vi "Desktop Main.vi"() -> ()   [LabVIEW 2018]
uses:
  Controls/Channel Settings.ctl
  Controls/Analog Input Selector.ctl
  Controls/Knob.ctl
  Controls/Vertical Position.ctl
  Controls/Time Selector.ctl
  Controls/Time Knob.ctl
  Controls/Instrument Control.ctl
  Controls/Acquisition Mode.ctl
  Controls/Measurements.ctl
  Controls/Channel Measurement String Control.ctl
  Controls/Options.ctl
  Controls/Channel.ctl
  Controls/Function Generator Control.ctl
  Program Files (x86)/National Instruments/LabVIEW 2018/ProjectTemplates/Source/myRIO/Oscilloscope/myRIO v1.1/Real-Time/Controls/Waveform Enum.ctl
  Program Files (x86)/National Instruments/LabVIEW 2018/ProjectTemplates/Source/myRIO/Oscilloscope/myRIO v1.1/Real-Time/Controls/Channel Selector.ctl
  Controls/Program Data.ctl
  Controls/Cursor Info.ctl
  Controls/Communication Cluster.ctl
  <vilib>/NI/STM/TCP/TCP Connection Info.ctl
  <vilib>/NI/STM/SubVIs/MetaDataElement.ctl
  Communication/Scope Data.ctl
  Program Files (x86)/National Instruments/LabVIEW 2018/ProjectTemplates/Source/myRIO/Oscilloscope/myRIO v1.1/Real-Time/Controls/Wave Parameters.ctl
  Controls/Channel Parameters.ctl
  Controls/FGen Desktop Configuration.ctl
  Controls/Measurement Selector.ctl
  Queue Library/User Event Action Enum.ctl
  Controls/Scope & FGen Parameters.ctl
  Controls/FGen FGV Enum.ctl
  Queue Library/Queue Library.lvlib
  <vilib>/NI/STM/NI STM.lvlib
panel:
  out "Acquiring?":bool
  out "Gen?":bool
  out "Sweep?":bool
  out "Scope Screen":waveform(dbl)[](graph)
  in  "Function Generator":T1 {"Vpeak (V)" min=0.0; "Frequency (Hz)" min=0.0}
  out "error out":errorcluster
  in  "Options":T4={"Enable\nCursors"=FALSE, "C1"=enum."CH 0", "C2"=enum."CH 0", "CH 0"=FALSE, "CH 1"=FALSE, "IP"="172.22.11.2"}
  out "Measurements":T6={"Channel 0"="Channel 0", "RMS 0"="RMS:", "Vp-p 0"="Vp-p:", "Freq 0"="Freq:", "Channel 1"="Channel 1", "RMS 1"="RMS:", "Vp-p 1"="Vp-p:", "Freq 1"="Freq:", "Cursors"="Cursors", "C1"="C1:", "C2"="C2:", "dT"="dT:"}
  in  "Acquisition Control":T8
  in  "Time":T10={"Time/Div"=6.0} {"Time/Div" min=0.0 max=16.0 step=1.0 scale=0.0..12.0}
  in  "Channel 1 Settings":T12={"Channel"=enum."AI 1", "Enable"=FALSE, "Volts/Div"=5, "Vertical Position (Div)"=0.0} {"Vertical Position (Div)" min=-5.0 max=5.0 step=0.1 scale=-5.0..5.0; "Volts/Div" min=0 max=8 step=1 scale=0.0..8.0}
  in  "Channel 0 Settings":T12={"Channel"=enum."AI 0", "Enable"=TRUE, "Volts/Div"=5, "Vertical Position (Div)"=0.0} {"Vertical Position (Div)" min=-5.0 max=5.0 step=0.1 scale=-5.0..5.0; "Volts/Div" min=0 max=8 step=1 scale=0.0..8.0}
  # "Scope & FGen for NI myRIO"
  # "Measurements"
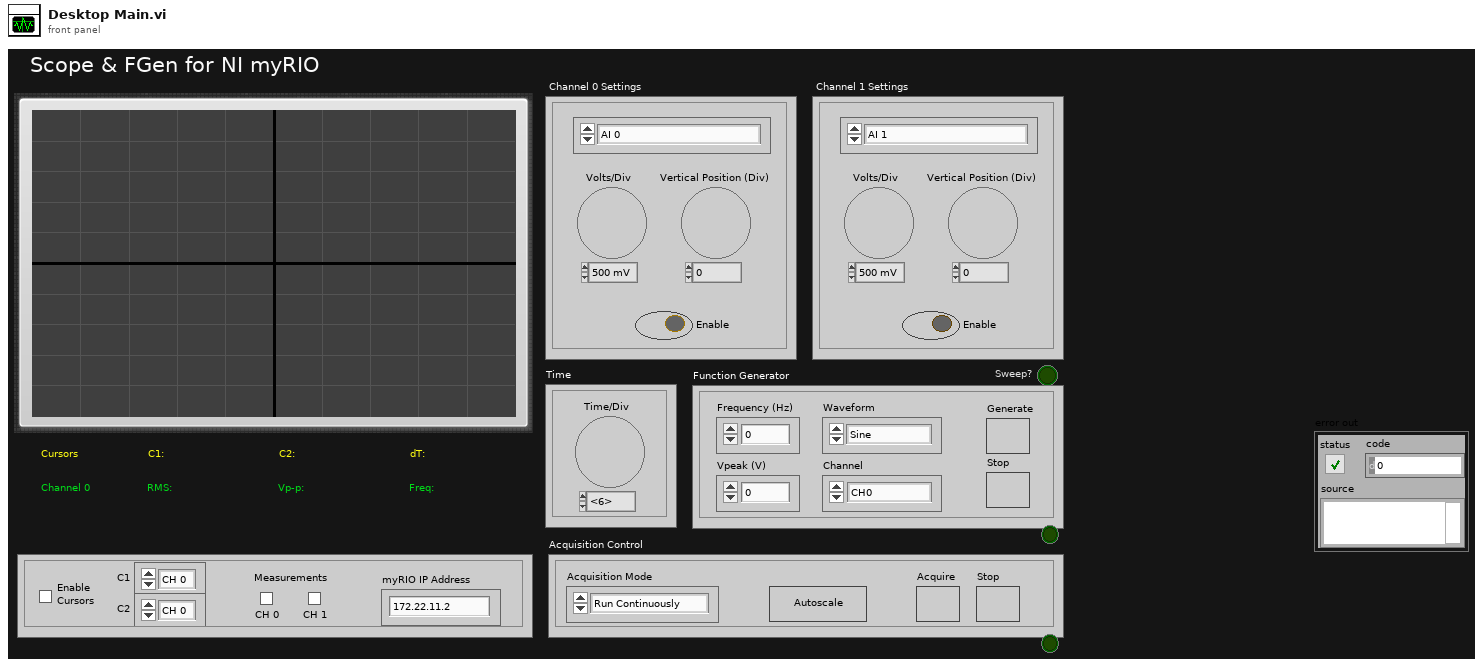
[diagram p1: front panel]
types:
  T1 = typedef "Function Generator Control.ctl" = cluster{"Frequency (Hz)":dbl, "Vpeak (V)":dbl, "Waveform":T2, "Channel":T3, "Generate":bool, "Stop":bool}
  T2 = typedef "Waveform Enum.ctl" = enum16{"Sine", "Square"}
  T3 = typedef "Channel Selector.ctl" = enum16{"CH0", "CH1"}
  T4 = typedef "Options.ctl" = cluster{"Enable\nCursors":bool, "C1":T5, "C2":T5, "CH 0":bool, "CH 1":bool, "IP":string}
  T5 = typedef "Channel.ctl" = enum16{"CH 0", "CH 1"}
  T6 = typedef "Measurements.ctl" = cluster{"Channel 0":T7, "RMS 0":T7, "Vp-p 0":T7, "Freq 0":T7, "Channel 1":T7, "RMS 1":T7, "Vp-p 1":T7, "Freq 1":T7, "Cursors":T7, "C1":T7, "C2":T7, "dT":T7}
  T7 = typedef "Channel Measurement String Control.ctl" = string
  T8 = typedef "Instrument Control.ctl" = cluster{"Acquisition Mode":T9, "Acquire":bool, "Stop":bool, "Autoscale":bool}
  T9 = typedef "Acquisition Mode.ctl" = enum16{"Run Continuously", "Run Once"}
  T10 = typedef "Time Selector.ctl" = cluster{"Time/Div":T11}
  T11 = typedef "Time Knob.ctl" = dbl
  T12 = typedef "Channel Settings.ctl" = cluster{"Channel":T13, "Enable":bool, "Volts/Div":T14, "Vertical Position (Div)":T15}
  T13 = typedef "Analog Input Selector.ctl" = enum16{"AI 0", "AI 1"}
  T14 = typedef "Knob.ctl" = i32
  T15 = typedef "Vertical Position.ctl" = dbl
  T16 = typedef "Queue Library.lvlib/User Event Action Enum.ctl" = enum16{"Initialize", "Generate", "Destroy"}
  T17 = typedef "Measurement Selector.ctl" = enum16{"CH0", "CH1", "Cursors"}
  T18 = typedef "Program Data.ctl" = cluster{"Measurements":T6, "C1":T19, "C2":T19, "Com":T20, "Continuous?":bool, "Scope Data":T23, "Wave Parameters":T24, "Acquire?":bool, "Measure Ref":refnum<vi>, "CH0":T12, "CH1":T12, "CH0 Params":T25, "CH1 Params":T25, "Time":T10, "dT":dbl, "FGen":T26}
  T19 = typedef "Cursor Info.ctl" = cluster{"Name":string, "X":dbl, "Y":dbl}
  T20 = typedef "Communication Cluster.ctl" = cluster{"Connection Info":T21, "Connected?":bool, "IP":string}
  T21 = typedef "NI STM.lvlib/TCP Connection Info.ctl" = cluster{"connection ID":refnum<k5>, "meta data":T22[]}
  T22 = typedef "NI STM.lvlib/MetaDataElement.ctl" = string
  T23 = typedef "Scope Data.ctl" = cluster{"AI0":dbl[], "AI1":dbl[]}
  T24 = typedef "Wave Parameters.ctl" = cluster{"Frequency (Hz)":dbl, "Phase offset (deg)":dbl, "Vpeak (V)":dbl, "Offset (V)":dbl, "Waveform":T2, "Channel":T3}
  T25 = typedef "Channel Parameters.ctl" = cluster{"V/Div":dbl, "Units":string}
  T26 = typedef "FGen Desktop Configuration.ctl" = cluster{"Offset (V)":dbl, "Enable Sweep":bool, "Start Frequency (Hz)":dbl, "Stop Frequency (Hz)":dbl, "Step (Hz)":dbl, "Step Interval (ms)":dbl, "Current Freq (Hz)":dbl, "Run":bool}
  T27 = typedef "FGen FGV Enum.ctl" = enum16{"Set", "Get"}
  T28 = typedef "Scope & FGen Parameters.ctl" = cluster{"Acquire?":bool, "Wave Parameters":T24, "Time":T10}
  T29 = typedef "State.ctl" = enum16{"Initialize", "Idle", "Start Scope", "Acquire", "Stop Scope", "Config FGen", "Start FGen", "Sweep FGen", "Stop FGen", "Plot", "Option Selection", "Channel 0 Selection", "Channel 1 Selection", "Update Cursors", "Update Measurements", "Time/Div", "Autoscale", "Stop", "Error"}
  T30 = cluster{"Cursor.Cursor Name":string, "Cursor.Cursor X":dbl, "Cursor.Cursor Y":dbl}
  T31 = cluster{"Cursor Name":string, "Cursor X":dbl, "Cursor Y":dbl}
  T32 = cluster{"Enable\nCursors":bool, "C1":bool, "C2":bool, "CH 0":bool, "CH 1":bool, "IP":bool}
  T33 = cluster{"Channel":bool, "Enable":bool, "Volts/Div":bool, "Vertical Position (Div)":bool}
  T34 = cluster{"Acquisition Mode":bool, "Acquire":bool, "Stop":bool, "Autoscale":bool}
  T35 = cluster{"Frequency (Hz)":bool, "Vpeak (V)":bool, "Waveform":bool, "Channel":bool, "Generate":bool, "Stop":bool}
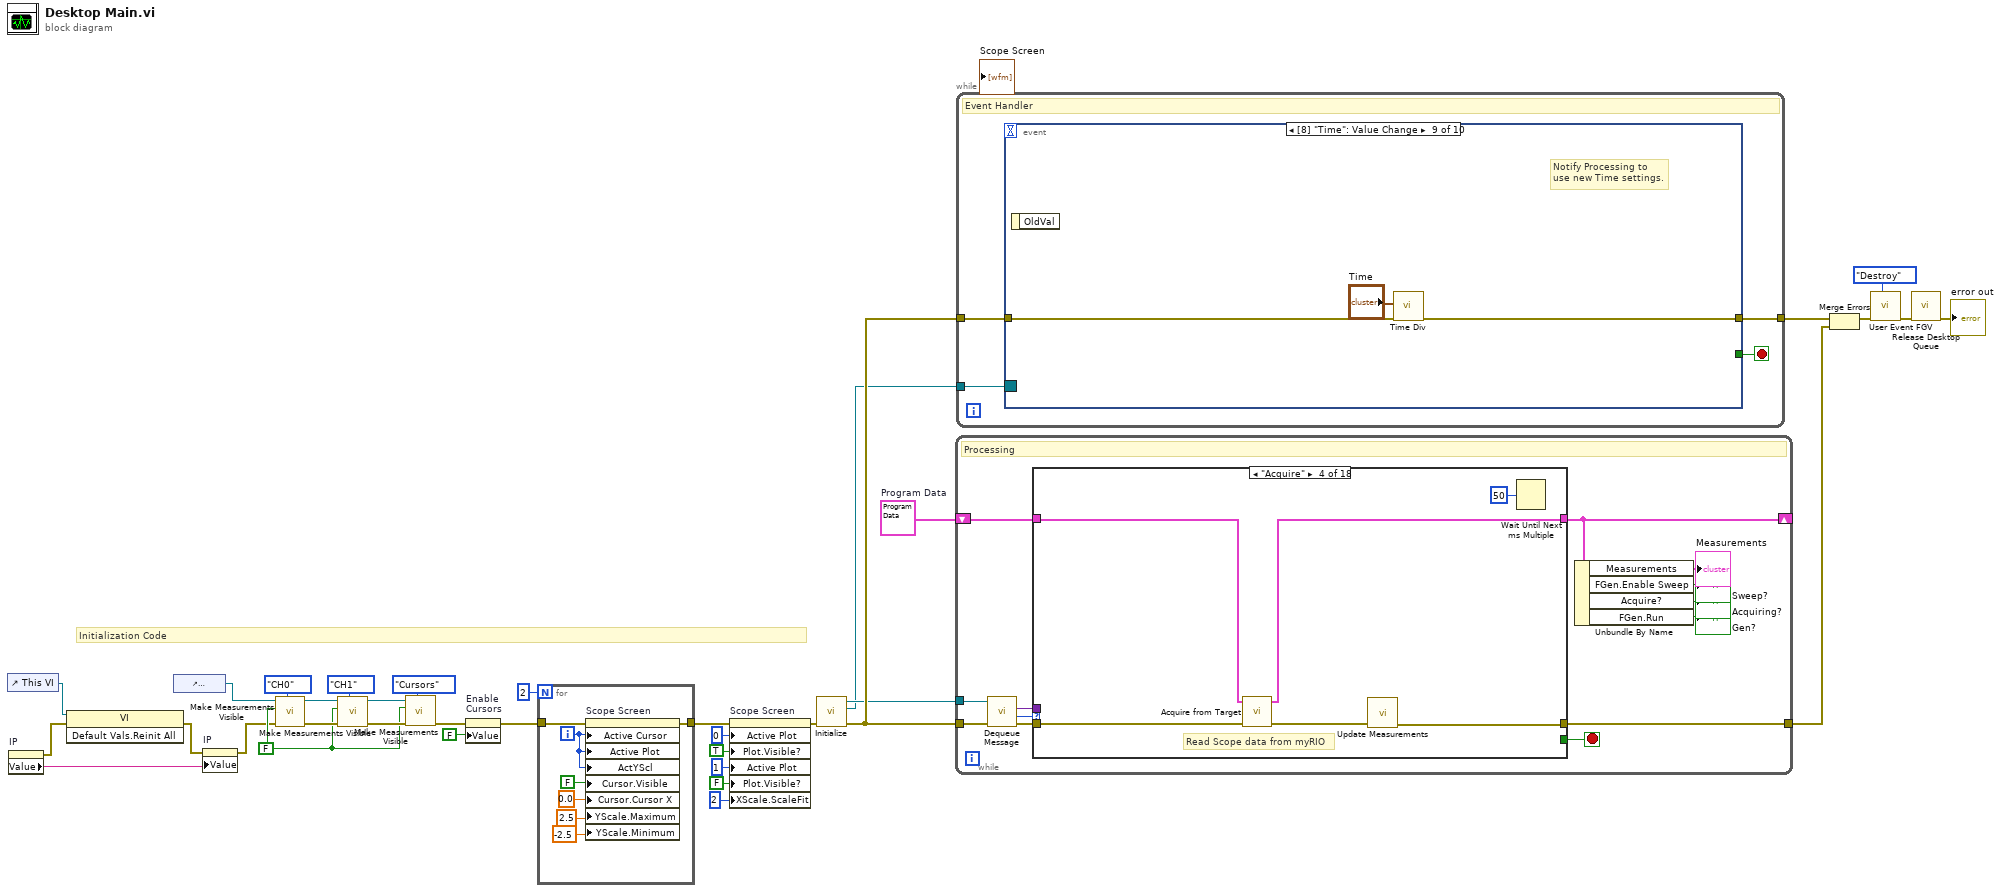
[diagram p0: block diagram]
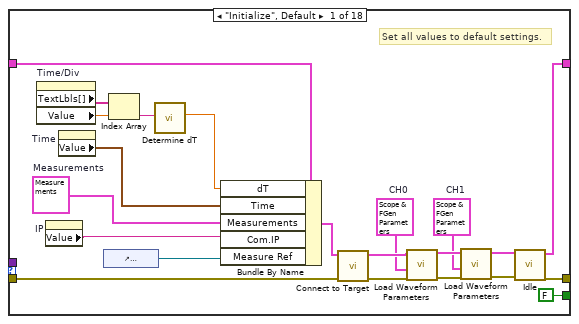
[diagram p2: hidden frame]
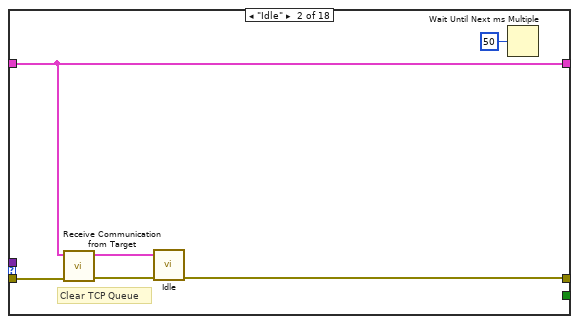
[diagram p3: hidden frame]
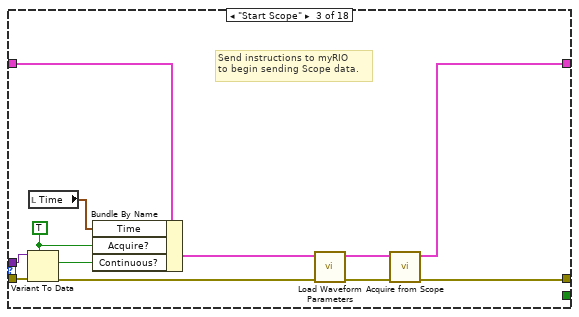
[diagram p4: hidden frame]
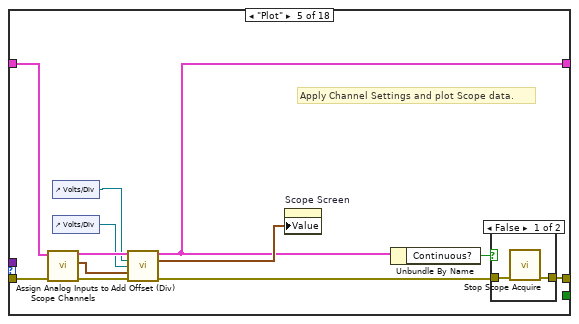
[diagram p5: hidden frame]
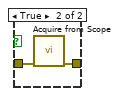
[diagram p6: hidden frame]
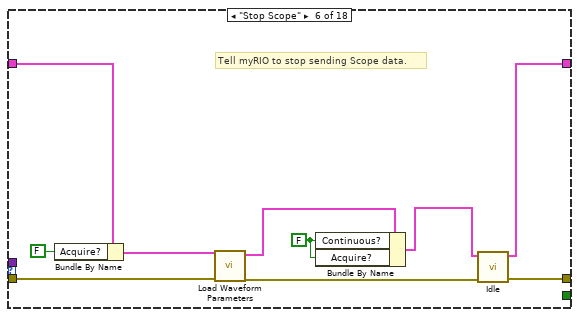
[diagram p7: hidden frame]
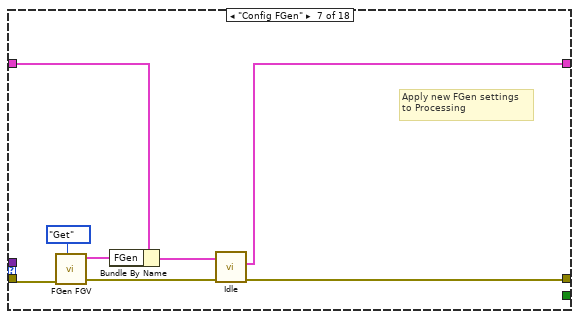
[diagram p8: hidden frame]
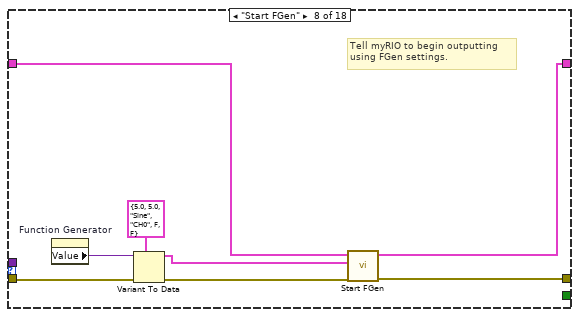
[diagram p9: hidden frame]
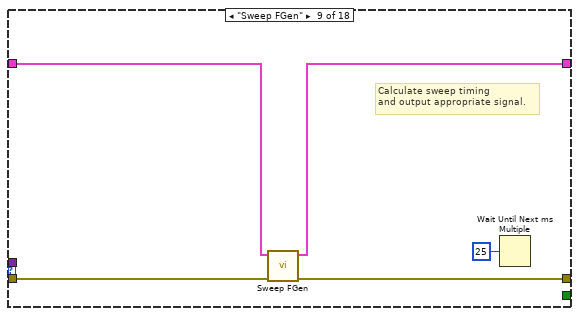
[diagram p10: hidden frame]
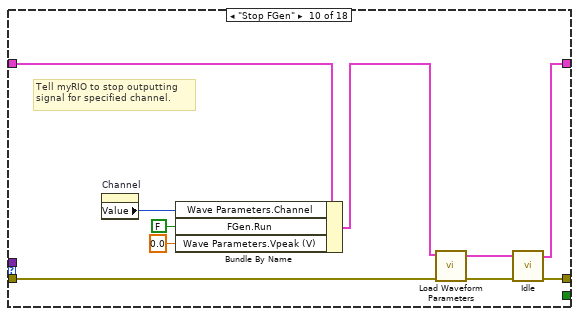
[diagram p11: hidden frame]
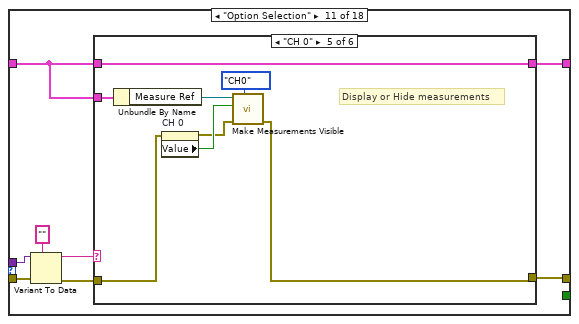
[diagram p12: hidden frame]
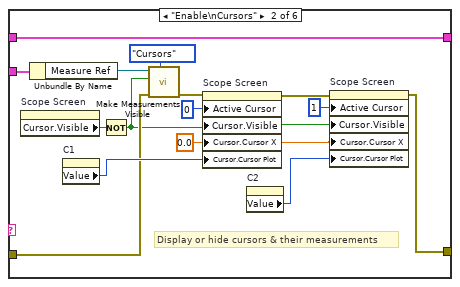
[diagram p14: hidden frame]
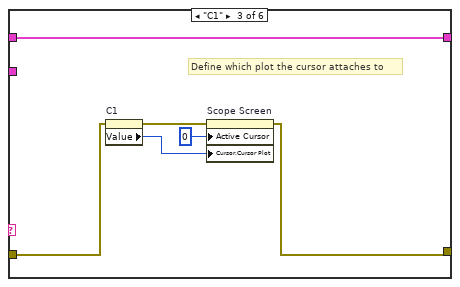
[diagram p15: hidden frame]
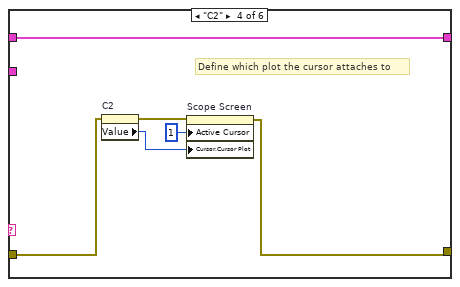
[diagram p16: hidden frame]
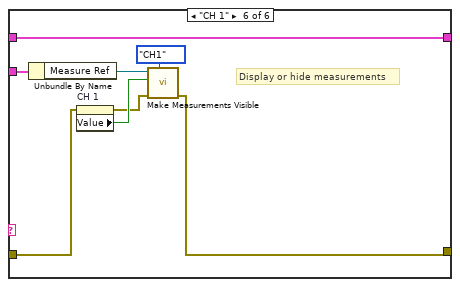
[diagram p17: hidden frame]
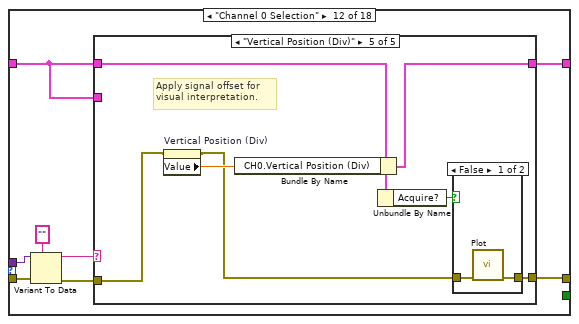
[diagram p18: hidden frame]
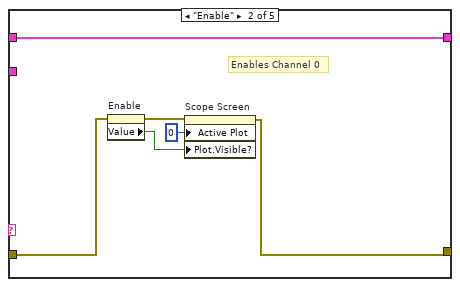
[diagram p20: hidden frame]
diagram:
  w17 = FALSE ("Visible?")
  w31 = T18 {"Measurements"={"Channel 0"="", "RMS 0"="", "Vp-p 0"="", "Freq 0"="", "Channel 1"="", "RMS 1"="", "Vp-p 1"="", "Freq 1"="", "Cursors"="", "C1"="", "C2"="", "dT"=""}, "C1"={"Name"="", "X"=0.0, "Y"=0.0}, "C2"={"Name"="", "X"=0.0, "Y"=0.0}, "Com"={"Connection Info"={"connection ID"=refnum, "meta data"=[]}, "Connected?"=FALSE, "IP"=""}, "Continuous?"=FALSE, "Scope Data"={"AI0"=[], "AI1"=[]}, "Wave Parameters"={"Frequency (Hz)"=0.0, "Phase offset (deg)"=0.0, "Vpeak (V)"=0.0, "Offset (V)"=0.0, "Waveform"=enum."Sine", "Channel"=enum."CH0"}, "Acquire?"=FALSE, "Measure Ref"=refnum, "CH0"={"Channel"=enum."AI 0", "Enable"=TRUE, "Volts/Div"=5, "Vertical Position (Div)"=0.0}, "CH1"={"Channel"=enum."AI 1", "Enable"=FALSE, "Volts/Div"=5, "Vertical Position (Div)"=0.0}, "CH0 Params"={"V/Div"=0.5, "Units"="V"}, "CH1 Params"={"V/Div"=0.5, "Units"="V"}, "Time"={"Time/Div"=0.0}, "dT"=0.0, "FGen"={"Offset (V)"=0.0, "Enable Sweep"=FALSE, "Start Frequency (Hz)"=0.0, "Stop Frequency (Hz)"=0.0, "Step (Hz)"=0.0, "Step Interval (ms)"=0.0, "Current Freq (Hz)"=0.0, "Run"=FALSE}}  # Program Data
  # "Initialization Code"
  n1 = control-ref of="This VI"() -> (w24:refnum<vi>)
  n2 = property on="IP" class="Str"() -> (error out=w2:errorcluster, "Value"=w1:string)  [unwired: 2 in, 1 out]
  n3 = invoke class="VI" method="Default Vals.Reinit All"(reference=w24, error in=w2) -> (error out=w4:errorcluster)  [unwired: 1 in, 2 out]
  n4 = control-ref of="Measurements"() -> (w16:refnum<vi>)
  n5 = property on="IP" class="Str"(error in=w4, "Value"=w1) -> (error out=w3:errorcluster)  [unwired: 1 in, 1 out]
  n6 = call "Make Measurements Visible.vi"("Item"=Measurement_Selector."CH0", "error in (no error)"=w3, "Visible?"=w17, "Measurements Ref"=w16) -> ("error out"=w23:errorcluster)  [unwired: 7 in]
  n7 = call "Make Measurements Visible.vi"("Item"=Measurement_Selector."CH1", "error in (no error)"=w23, "Visible?"=w17, "Measurements Ref"=w16) -> ("error out"=w20:errorcluster)  [unwired: 7 in]
  n8 = call "Make Measurements Visible.vi"("Item"=Measurement_Selector."Cursors", "error in (no error)"=w20, "Visible?"=w17, "Measurements Ref"=w16) -> ("error out"=w19:errorcluster)  [unwired: 7 in]
  n9 = property on="Enable\nCursors" class="Bool (strict)"(error in=w19, "Value"=FALSE) -> (error out=w25:errorcluster)  [unwired: 1 in, 1 out]
  n10 = for {
    N: 2 -> [_]
    tunnel: w25 -> [w38]
    tunnel: [w37] -> w11
    i -> [w36]
    n11 = property on="Scope Screen" class="WFGraph (strict)"(error in=w38, "Active Cursor"=w36, "Active Plot"=w36, "ActYScl"=w36, "Cursor.Visible"=FALSE, "Cursor.Cursor X"=0.0 ("Cursor.Cursor Position:Cursor X"), "YScale.Maximum"=2.5 ("Y Scale.Range:Maximum"), "YScale.Minimum"=-2.5 ("Y Scale.Range:Minimum")) -> (error out=w37:errorcluster)  [unwired: 1 in, 1 out]
  }
  n12 = property on="Scope Screen" class="WFGraph (strict)"(error in=w11, "Active Plot"=u32 0, "Plot.Visible?"=TRUE ("Plot.Visible"), "Active Plot"=u32 1, "Plot.Visible?"=FALSE ("Plot.Visible"), "XScale.ScaleFit"=u8 2 ("X Scale.Scale Fit")) -> (error out=w6:errorcluster)  [unwired: 1 in, 1 out]
  n13 = call "Initialize.vi"("error in (no error)"=w6) -> ("error out"=w30:errorcluster, "User Event Out"=w10:refnum<event-registration>, "queue out"=w29:refnum<queue>)  [unwired: 8 in]
  n14 = while {
    tunnel: w29 -> [w43]
    tunnel: w30 -> [w53]
    tunnel: [w48] -> w32
    shift-right: [w46] -> _
    shift-left: w31 -> [w47]
    stop <- w50 stop-if-true
    # "Processing"
    n15 = call "Dequeue Message.vi"("error in (no error)"=w53, "queue in"=w43) -> ("error out"=w49:errorcluster, "State"=w52:T29, "Data"=w51:variant)  [unwired: 6 in, 1 out]
    n16 = case shown="\"Acquire\"" w52 {
      tunnel: w51 -> [_ _ w91 _ _ _ _ _ _ _ w162 w215 w260 _ w333 w346 _ _]
      tunnel: [FALSE _ _ _ _ _ _ _ _ _ _ _ _ FALSE FALSE _ _ TRUE] -> w50
      tunnel: w49 -> [w72 w81 w92 w97 w107 w123 w131 w140 w145 w153 w163 w216 w261 w306 w334 w347 w380 w391]
      tunnel: [w67 w78 w86 w93 w110 w118 w125 w139 w143 w155 w158 w211 w256 w311 w327 w341 w377 w388] -> w48
      tunnel: w47 -> [w74 w80 w84 w96 w108 w121 w132 w133 w144 w152 w157 w210 w255 w308 w330 w338 w379 w387]
      tunnel: [w66 w80 w90 w95 w101 w115 w126 w138 w142 w148 w156 w209 w254 w300 w329 w339 w375 w386] -> w46
      frame "Initialize", Default {
        w54 = T28 {"Acquire?"=FALSE, "Wave Parameters"={"Frequency (Hz)"=0.0, "Phase offset (deg)"=0.0, "Vpeak (V)"=0.0, "Offset (V)"=0.0, "Waveform"=enum."Sine", "Channel"=enum."CH1"}, "Time"={"Time/Div"=9.0}}  # CH1
        w68 = T28 {"Acquire?"=FALSE, "Wave Parameters"={"Frequency (Hz)"=0.0, "Phase offset (deg)"=0.0, "Vpeak (V)"=0.0, "Offset (V)"=0.0, "Waveform"=enum."Sine", "Channel"=enum."CH0"}, "Time"={"Time/Div"=9.0}}  # CH0
        w73 = T6 {"Channel 0"="Channel 0", "RMS 0"="RMS:", "Vp-p 0"="Vp-p:", "Freq 0"="Freq:", "Channel 1"="Channel 1", "RMS 1"="RMS:", "Vp-p 1"="Vp-p:", "Freq 1"="Freq:", "Cursors"="Cursors", "C1"="C1:", "C2"="C2:", "dT"="dT:"}  # Measurements
        # "Set all values to default settings."
        n17 = property on="Time/Div" class="Knob (strict)"() -> ("TextLbls[]"=w63:string[], "Value"=w62:T11)  [unwired: 2 in, 2 out]
        n18 = property on="IP" class="Str"() -> ("Value"=w59:string)  [unwired: 2 in, 2 out]
        n19 = property on="Time" class="Clust (strict)"() -> ("Value"=w64:T10)  [unwired: 2 in, 2 out]
        n20 = control-ref of="Measurements"() -> (w65:refnum<vi>)
        n21 = Index Array(array=w63, index=w62) -> (element=w61:string)
        n22 = call "Determine dT.vi"("Time/Div"=w61) -> ("dT"=w60:dbl)  [unwired: 6 in, 4 out]
        n23 = Bundle By Name(cluster=w74, "dT"=w60, "Time"=w64, "Measurements"=w73, "Com.IP"=w59, "Measure Ref"=w65) -> (w71:T18)
        n24 = call "Connect to Target.vi"("error in"=w72, "Program Data"=w71) -> ("error out"=w70:errorcluster, "Program Data Out"=w69:T18)  [unwired: 8 in]
        n25 = call "Load Waveform Parameters.vi"("error in (no error)"=w70, "Params"=w68, "Program Data"=w69) -> ("error out"=w58:errorcluster, "Program Data Out"=w56:T18)  [unwired: 7 in]
        n26 = call "Load Waveform Parameters.vi"("error in (no error)"=w58, "Params"=w54, "Program Data"=w56) -> ("error out"=w57:errorcluster, "Program Data Out"=w55:T18)  [unwired: 7 in]
        n27 = call "Idle.vi"("error in (no error)"=w57, "Program Data"=w55) -> ("error out"=w67:errorcluster, "Program Data Out"=w66:T18)  [unwired: 7 in, 1 out]
      }
      frame "Idle" {
        # "Clear TCP Queue"
        n28 = call "Receive Communication from Target.vi"("error in (no error)"=w81, "Program Data"=w80) -> ("error out"=w79:errorcluster, "Program Data Out"=w76:T18)  [unwired: 8 in]
        n29 = call "Idle.vi"("error in (no error)"=w79, "Program Data"=w76) -> ("error out"=w78:errorcluster)  [unwired: 7 in, 2 out]
        n30 = Wait Until Next ms Multiple(millisecond multiple=u32 50) -> ()  [unwired: 1 out]
      }
      frame "Start Scope" {
        w85 = TRUE
        # "Send instructions to myRIO\nto begin sending Scope data."
        n31 = Variant To Data(error in=w92, type=w85, Variant=w91) -> (data=w89:bool, error out=w88:errorcluster)
        n32 = local read "Time"() -> (w82:T10)
        n33 = Bundle By Name(cluster=w84, "Time"=w82, "Acquire?"=w85, "Continuous?"=w89) -> (w83:T18)
        n34 = call "Load Waveform Parameters.vi"("error in (no error)"=w88, "Program Data"=w83) -> ("error out"=w87:errorcluster, "Program Data Out"=w90:T18)  [unwired: 8 in]
        n35 = call "Acquire from Scope.vi"("error in (no error)"=w87) -> ("error out"=w86:errorcluster)  [unwired: 9 in, 1 out]
      }
      frame "Acquire" {
        # "Read Scope data from myRIO"
        n36 = call "Acquire from Target.vi"("error in (no error)"=w97, "Program Data"=w96) -> ("error out"=w94:errorcluster, "Program Data Out"=w95:T18)  [unwired: 8 in]
        n37 = call "Update Measurements.vi"("error in (no error)"=w94) -> ("error out"=w93:errorcluster)  [unwired: 9 in, 1 out]
        n38 = Wait Until Next ms Multiple(millisecond multiple=u32 50) -> ()  [unwired: 1 out]
      }
      frame "Plot" {
        # "Apply Channel Settings and plot Scope data."
        n39 = call "Assign Analog Inputs to Scope Channels.vi"("error in (no error)"=w107, "Program Data"=w108) -> ("error out"=w105:errorcluster, "Scope Data"=w102:waveform(dbl)[], "Program Data Out"=w106:T18)  [unwired: 7 in]
        n40 = control-ref of="Volts/Div"() -> (w100:refnum<vi>)
        n41 = control-ref of="Volts/Div"() -> (w99:refnum<vi>)
        n42 = call "Add Offset (Div).vi"("Program Data"=w106, "CH 0 in"=w100, "CH 1 in"=w99, "Scope Data"=w102, "error in (no error)"=w105) -> ("Program Data Out"=w101:T18, "Plots"=w103:waveform(dbl)[], "error out"=w104:errorcluster)  [unwired: 8 in]
        n43 = property on="Scope Screen" class="WFGraph (strict)"("Value"=w103) -> ()  [unwired: 2 in, 2 out]
        n44 = Unbundle By Name(w101) -> ("Continuous?"=w109:bool)
        n45 = case shown="False" w109 {
          tunnel: [w112 w114] -> w110
          tunnel: w104 -> [w111 w113]
          frame False {
            n46 = call "Stop Scope Acquire.vi"("error in (no error)"=w111) -> ("error out"=w112:errorcluster)  [unwired: 9 in, 1 out]
          }
          frame True {
            n47 = call "Acquire from Scope.vi"("error in (no error)"=w113) -> ("error out"=w114:errorcluster)  [unwired: 9 in, 1 out]
          }
        }
      }
      frame "Stop Scope" {
        w124 = FALSE ("Continuous?")
        # "Tell myRIO to stop sending Scope data."
        n48 = Bundle By Name(cluster=w121, "Acquire?"=FALSE) -> (w120:T18)
        n49 = call "Load Waveform Parameters.vi"("error in (no error)"=w123, "Program Data"=w120) -> ("error out"=w117:errorcluster, "Program Data Out"=w122:T18)  [unwired: 8 in]
        n50 = Bundle By Name(cluster=w122, "Continuous?"=w124, "Acquire?"=w124) -> (w116:T18)
        n51 = call "Idle.vi"("error in (no error)"=w117, "Program Data"=w116) -> ("error out"=w118:errorcluster, "Program Data Out"=w115:T18)  [unwired: 7 in, 1 out]
      }
      frame "Config FGen" {
        # "Apply new FGen settings\nto Processing"
        n52 = call "FGen FGV.vi"("Action"=FGen_FGV_Enum."Get", "error in (no error)"=w131) -> ("error out"=w128:errorcluster, "FGen Out"=w129:T26)  [unwired: 8 in]
        n53 = Bundle By Name(cluster=w132, "FGen"=w129) -> (w127:T18)
        n54 = call "Idle.vi"("error in (no error)"=w128, "Program Data"=w127) -> ("error out"=w125:errorcluster, "Program Data Out"=w126:T18)  [unwired: 7 in, 1 out]
      }
      frame "Start FGen" {
        # "Tell myRIO to begin outputting\nusing FGen settings."
        n55 = property on="Function Generator" class="Clust"() -> ("Value"=w137:variant)  [unwired: 2 in, 2 out]
        n56 = Variant To Data(error in=w140, type=T1 {"Frequency (Hz)"=5.0, "Vpeak (V)"=5.0, "Waveform"=enum."Sine", "Channel"=enum."CH0", "Generate"=FALSE, "Stop"=FALSE} ("Function Generator 2"), Variant=w137) -> (data=w134:T1, error out=w136:errorcluster)
        n57 = call "Start FGen.vi"("error in (no error)"=w136, "Function Generator in"=w134, "Program Data"=w133) -> ("error out"=w139:errorcluster, "Program Data Out"=w138:T18)  [unwired: 7 in]
      }
      frame "Sweep FGen" {
        # "Calculate sweep timing\nand output appropriate signal."
        n58 = call "Sweep FGen.vi"("error in (no error)"=w145, "Program Data in"=w144) -> ("error out"=w143:errorcluster, "Program Data out"=w142:T18)  [unwired: 8 in]
        n59 = Wait Until Next ms Multiple(millisecond multiple=u32 25) -> ()  [unwired: 1 out]
      }
      frame "Stop FGen" {
        # "Tell myRIO to stop outputting\nsignal for specified channel."
        n60 = property on="Channel" class="Enum (strict)"() -> ("Value"=w146:T3)  [unwired: 2 in, 2 out]
        n61 = Bundle By Name(cluster=w152, "Wave Parameters.Channel"=w146, "FGen.Run"=FALSE, "Wave Parameters.Vpeak (V)"=0.0) -> (w151:T18)
        n62 = call "Load Waveform Parameters.vi"("error in (no error)"=w153, "Program Data"=w151) -> ("error out"=w154:errorcluster, "Program Data Out"=w149:T18)  [unwired: 8 in]
        n63 = call "Idle.vi"("error in (no error)"=w154, "Program Data"=w149) -> ("error out"=w155:errorcluster, "Program Data Out"=w148:T18)  [unwired: 7 in, 1 out]
      }
      frame "Option Selection" {
        n64 = Variant To Data(error in=w163, type="", Variant=w162) -> (data=w160:string, error out=w159:errorcluster)
        n65 = case shown="\"CH 0\"" w160 {
          tunnel: w159 -> [w165 w171 w183 w189 w196 w203]
          tunnel: [w165 w173 w182 w188 w193 w204] -> w158
          tunnel: w157 -> [_ w172 _ _ w197 w205]
          tunnel: w157 -> [w164 w166 w181 w187 w200 w208]
          tunnel: [w164 w166 w181 w187 w200 w208] -> w156
          frame "False", Default {
          }
          frame "Enable\nCursors" {
            w175 = 0.0 ("Cursor.Cursor Position:Cursor X")
            # "Display or hide cursors & their measurements"
            n66 = property on="Scope Screen" class="WFGraph (strict)"() -> ("Cursor.Visible"=w180:bool)  [unwired: 2 in, 2 out]
            n67 = Unbundle By Name(w172) -> ("Measure Ref"=w169:refnum<vi>)
            n68 = property on="C1" class="Enum (strict)"() -> ("Value"=w178:T5)  [unwired: 2 in, 2 out]
            n69 = Not(x=w180) -> (.not. x?=w168:bool)
            n70 = call "Make Measurements Visible.vi"("Item"=Measurement_Selector."Cursors", "error in (no error)"=w171, "Visible?"=w168, "Measurements Ref"=w169) -> ("error out"=w170:errorcluster)  [unwired: 7 in]
            n71 = property on="Scope Screen" class="WFGraph (strict)"(error in=w170, "Active Cursor"=u32 0, "Cursor.Visible"=w168, "Cursor.Cursor X"=w175, "Cursor.Cursor Plot"=w178) -> (error out=w177:errorcluster)  [unwired: 1 in, 1 out]
            n72 = property on="C2" class="Enum (strict)"() -> ("Value"=w174:T5)  [unwired: 2 in, 2 out]
            n73 = property on="Scope Screen" class="WFGraph (strict)"(error in=w177, "Active Cursor"=u32 1, "Cursor.Visible"=w168, "Cursor.Cursor X"=w175, "Cursor.Cursor Plot"=w174) -> (error out=w173:errorcluster)  [unwired: 1 in, 1 out]
          }
          frame "C1" {
            # "Define which plot the cursor attaches to"
            n74 = property on="C1" class="Enum (strict)"(error in=w183) -> (error out=w185:errorcluster, "Value"=w184:T5)  [unwired: 1 in, 1 out]
            n75 = property on="Scope Screen" class="WFGraph (strict)"(error in=w185, "Active Cursor"=u32 0, "Cursor.Cursor Plot"=w184) -> (error out=w182:errorcluster)  [unwired: 1 in, 1 out]
          }
          frame "C2" {
            # "Define which plot the cursor attaches to"
            n76 = property on="C2" class="Enum (strict)"(error in=w189) -> (error out=w192:errorcluster, "Value"=w190:T5)  [unwired: 1 in, 1 out]
            n77 = property on="Scope Screen" class="WFGraph (strict)"(error in=w192, "Active Cursor"=u32 1, "Cursor.Cursor Plot"=w190) -> (error out=w188:errorcluster)  [unwired: 1 in, 1 out]
          }
          frame "CH 0" {
            # "Display or Hide measurements"
            n78 = Unbundle By Name(w197) -> ("Measure Ref"=w199:refnum<vi>)
            n79 = property on="CH 0" class="Bool (strict)"(error in=w196) -> (error out=w194:errorcluster, "Value"=w195:bool)  [unwired: 1 in, 1 out]
            n80 = call "Make Measurements Visible.vi"("Item"=Measurement_Selector."CH0", "error in (no error)"=w194, "Visible?"=w195, "Measurements Ref"=w199) -> ("error out"=w193:errorcluster)  [unwired: 7 in]
          }
          frame "CH 1" {
            # "Display or hide measurements"
            n81 = Unbundle By Name(w205) -> ("Measure Ref"=w207:refnum<vi>)
            n82 = property on="CH 1" class="Bool (strict)"(error in=w203) -> (error out=w201:errorcluster, "Value"=w202:bool)  [unwired: 1 in, 1 out]
            n83 = call "Make Measurements Visible.vi"("Item"=Measurement_Selector."CH1", "error in (no error)"=w201, "Visible?"=w202, "Measurements Ref"=w207) -> ("error out"=w204:errorcluster)  [unwired: 7 in]
          }
        }
      }
      frame "Channel 0 Selection" {
        n84 = Variant To Data(error in=w216, type="", Variant=w215) -> (data=w213:string, error out=w212:errorcluster)
        n85 = case shown="\"Vertical Position (Div)\"" w213 {
          tunnel: w212 -> [w218 w221 w232 w242 w249]
          tunnel: [w218 w223 w231 w241 w244] -> w211
          tunnel: w210 -> [_ _ _ _ _]
          tunnel: w210 -> [w217 w222 w229 w239 w247]
          tunnel: [w217 w222 w228 w240 w250] -> w209
          frame "False", Default {
          }
          frame "Enable" {
            # "Enables Channel 0"
            n86 = property on="Enable" class="Bool (strict)"(error in=w221) -> (error out=w220:errorcluster, "Value"=w219:bool)  [unwired: 1 in, 1 out]
            n87 = property on="Scope Screen" class="WFGraph (strict)"(error in=w220, "Active Plot"=u32 0 ("Active Cursor"), "Plot.Visible?"=w219) -> (error out=w223:errorcluster)  [unwired: 1 in, 1 out]
          }
          frame "Volts/Div" {
            # "Adjust plot range according to Volts/Div"
            n88 = property on="Volts/Div" class="Knob (strict)"(error in=w232) -> (error out=w235:errorcluster, "TextLbls[]"=w238:string[], "Value"=w225:T14)  [unwired: 1 in, 1 out]
            n89 = Index Array(array=w238, index=w225) -> (element=w237:string)
            n90 = call "Determine Y Scale Limits.vi"("error in (no error)"=w235, "Volts/Div"=w237) -> ("error out"=w236:errorcluster, "Y Min"=w233:dbl, "Y Max"=w234:dbl, "Volts/Div"=w227:dbl, "Units"=w226:string)  [unwired: 5 in]
            n91 = Bundle By Name(cluster=w229, "CH0.Volts/Div"=w225, "CH0 Params.Units"=w226, "CH0 Params.V/Div"=w227) -> (w228:T18)
            n92 = property on="Scope Screen" class="WFGraph (strict)"(error in=w236, "ActYScl"=0 ("Active Y Scale"), "YScale.Maximum"=w234, "YScale.Minimum"=w233) -> (error out=w231:errorcluster)  [unwired: 1 in, 1 out]
          }
          frame "Channel" {
            # "Define which Analog Input\nthe Channel refers to."
            n93 = property on="Channel" class="Enum (strict)"(error in=w242) -> (error out=w241:errorcluster, "Value"=w243:T13)  [unwired: 1 in, 1 out]
            n94 = Bundle By Name(cluster=w239, "CH0.Channel"=w243) -> (w240:T18)
          }
          frame "Vertical Position (Div)" {
            # "Apply signal offset for \nvisual interpretation."
            n95 = property on="Vertical Position (Div)" class="Knob (strict)"(error in=w249) -> (error out=w245:errorcluster, "Value"=w248:T15)  [unwired: 1 in, 1 out]
            n96 = Bundle By Name(cluster=w247, "CH0.Vertical Position (Div)"=w248) -> (w250:T18)
            n97 = Unbundle By Name(w247) -> ("Acquire?"=w246:bool)
            n98 = case shown="False" w246 {
              tunnel: w245 -> [w252 w253]
              tunnel: [w251 w253] -> w244
              frame False {
                n99 = call "Plot.vi"("error in (no error)"=w252) -> ("error out"=w251:errorcluster)  [unwired: 9 in, 1 out]
              }
              frame True {
              }
            }
          }
        }
      }
      frame "Channel 1 Selection" {
        n100 = Variant To Data(error in=w261, type="", Variant=w260) -> (data=w258:string, error out=w257:errorcluster)
        n101 = case shown="\"Vertical Position (Div)\"" w258 {
          tunnel: w257 -> [w263 w267 w278 w286 w294]
          tunnel: [w263 w269 w279 w285 w290] -> w256
          tunnel: w255 -> [_ _ _ _ _]
          tunnel: w255 -> [w262 w268 w274 w287 w295]
          tunnel: [w262 w268 w273 w288 w289] -> w254
          frame "False", Default {
          }
          frame "Enable" {
            # "Enables Channel 1"
            n102 = property on="Enable" class="Bool (strict)"(error in=w267) -> (error out=w266:errorcluster, "Value"=w265:bool)  [unwired: 1 in, 1 out]
            n103 = property on="Scope Screen" class="WFGraph (strict)"(error in=w266, "Active Plot"=u32 1 ("Active Cursor"), "Plot.Visible?"=w265) -> (error out=w269:errorcluster)  [unwired: 1 in, 1 out]
          }
          frame "Volts/Div" {
            # "Adjust plot range according to Volts/Div"
            n104 = property on="Volts/Div" class="Knob (strict)"(error in=w278) -> (error out=w276:errorcluster, "TextLbls[]"=w277:string[], "Value"=w270:T14)  [unwired: 1 in, 1 out]
            n105 = Index Array(array=w277, index=w270) -> (element=w283:string)
            n106 = call "Determine Y Scale Limits.vi"("error in (no error)"=w276, "Volts/Div"=w283) -> ("error out"=w282:errorcluster, "Y Min"=w280:dbl, "Y Max"=w281:dbl, "Volts/Div"=w272:dbl, "Units"=w271:string)  [unwired: 5 in]
            n107 = Bundle By Name(cluster=w274, "CH1.Volts/Div"=w270, "CH1 Params.Units"=w271, "CH1 Params.V/Div"=w272) -> (w273:T18)
            n108 = property on="Scope Screen" class="WFGraph (strict)"(error in=w282, "ActYScl"=1 ("Active Y Scale"), "YScale.Maximum"=w281, "YScale.Minimum"=w280) -> (error out=w279:errorcluster)  [unwired: 1 in, 1 out]
          }
          frame "Channel" {
            # "Define which Analog Input\nthe Channel refers to."
            n109 = property on="Channel" class="Enum (strict)"(error in=w286) -> (error out=w285:errorcluster, "Value"=w284:T13)  [unwired: 1 in, 1 out]
            n110 = Bundle By Name(cluster=w287, "CH1.Channel"=w284) -> (w288:T18)
          }
          frame "Vertical Position (Div)" {
            # "Apply signal offset for \nvisual interpretation."
            n111 = property on="Vertical Position (Div)" class="Knob (strict)"(error in=w294) -> (error out=w291:errorcluster, "Value"=w293:T15)  [unwired: 1 in, 1 out]
            n112 = Bundle By Name(cluster=w295, "CH1.Vertical Position (Div)"=w293) -> (w289:T18)
            n113 = Unbundle By Name(w289) -> ("Acquire?"=w292:bool)
            n114 = case shown="False" w292 {
              tunnel: w291 -> [w297 w298]
              tunnel: [w296 w298] -> w290
              frame False {
                n115 = call "Plot.vi"("error in (no error)"=w297) -> ("error out"=w296:errorcluster)  [unwired: 9 in, 1 out]
              }
              frame True {
              }
            }
          }
        }
      }
      frame "Update Measurements" {
        # "Calculate all measurements for each channel.\nUpdate cursor values and calculations."
        n116 = property on="Time/Div" class="Knob (strict)"() -> ("TextLbls[]"=w310:string[], "Value"=w309:T11)  [unwired: 2 in, 2 out]
        n117 = Index Array(array=w310, index=w309) -> (element=w301:string)
        n118 = call "Determine dT.vi"("error in (no error)"=w306, "Time/Div"=w301, "Program Data"=w308) -> ("error out"=w305:errorcluster, "Program Data Out"=w307:T18)  [unwired: 4 in, 3 out]
        n119 = call "Calculate Measurements.vi"("error in (no error)"=w305, "Program Data"=w307) -> ("error out"=w304:errorcluster, "Program Data Out"=w303:T18)  [unwired: 8 in]
        n120 = for {
          N: 2 -> [_]
          tunnel: w304 -> [w318]
          tunnel: [w317] -> w302
          tunnel: w301 -> [w314]
          shift-right: [w316] -> w300
          shift-left: w303 -> [w313]
          i -> [w322]
          n121 = property on="Scope Screen" class="WFGraph (strict)"("Active Cursor"=w322) -> ("Cursor.Cursor Name"=w320:string, "Cursor.Cursor X"=w321:dbl, "Cursor.Cursor Y"=w319:dbl)  [unwired: 2 in, 2 out]
          n122 = Bundle("Cursor.Cursor Name"=w320, "Cursor.Cursor X"=w321, "Cursor.Cursor Y"=w319) -> (w315:T30)  [unwired: 1 in]
          n123 = call "Update Cursor Indicator.vi"("error in (no error)"=w318, "Cursor Info"=w315, "Time/Div"=w314, "Program Data"=w313) -> ("error out"=w317:errorcluster, "Program Data Out"=w316:T18)  [unwired: 6 in]
        }
        n124 = call "Plot.vi"("error in (no error)"=w302) -> ("error out"=w311:errorcluster)  [unwired: 9 in, 1 out]
      }
      frame "Update Cursors" {
        # "Update cursor values and calculations."
        n125 = property on="Time/Div" class="Knob (strict)"() -> ("TextLbls[]"=w325:string[], "Value"=w324:T11)  [unwired: 2 in, 2 out]
        n126 = Variant To Data(error in=w334, type=T19 {"Name"="", "X"=0.0, "Y"=0.0} ("output cluster"), Variant=w333) -> (data=w326:T19, error out=w328:errorcluster)
        n127 = Index Array(array=w325, index=w324) -> (element=w323:string)
        n128 = call "Update Cursor Indicator.vi"("error in (no error)"=w328, "Cursor Info"=w326, "Time/Div"=w323, "Program Data"=w330) -> ("error out"=w327:errorcluster, "Program Data Out"=w329:T18)  [unwired: 6 in]
      }
      frame "Time/Div" {
        n129 = Unbundle By Name(w338) -> ("Acquire?"=w335:bool)
        n130 = Variant To Data(error in=w347, type=T10 {"Time/Div"=9.0} ("Time 2"), Variant=w346) -> (data=w343:T10, error out=w337:errorcluster)
        n131 = case shown="False" w335 {
          tunnel: [w356 w369] -> w344
          tunnel: w343 -> [_ w368]
          tunnel: w338 -> [w351 w362]
          tunnel: w337 -> [w355 w361]
          tunnel: [w357 w360] -> w336
          frame False {
            # "Adjust plot range and acquisition\nsettings based on specified \nTime/Div."
            n132 = property on="Scope Screen" class="WFGraph (strict)"(error in=w355, "XScale.ScaleFit"=u8 0 ("X Scale.Scale Fit")) -> (error out=w353:errorcluster)  [unwired: 1 in, 1 out]
            n133 = control-ref of="Scope Screen"() -> (w349:refnum<vi>)
            n134 = property on="Time/Div" class="Knob (strict)"(error in=w353) -> (error out=w352:errorcluster, "TextLbls[]"=w354:string[], "Value"=w348:T11)  [unwired: 1 in, 1 out]
            n135 = Index Array(array=w354, index=w348) -> (element=w350:string)
            n136 = call "Static Time-Div Change.vi"("error in (no error)"=w352, "WFGraph Refnum"=w349, "Time/Div"=w350, "Program Data"=w351) -> ("error out"=w357:errorcluster, "Program Data Out"=w356:T18)  [unwired: 6 in]
          }
          frame True {
            n137 = property on="Scope Screen" class="WFGraph (strict)"("XScale.ScaleFit"=u8 2 ("X Scale.Scale Fit")) -> ()  [unwired: 2 in, 2 out]
            n138 = property on="Time/Div" class="Knob (strict)"() -> ("TextLbls[]"=w366:string[], "Value"=w365:T11)  [unwired: 2 in, 2 out]
            n139 = Index Array(array=w366, index=w365) -> (element=w363:string)
            n140 = call "Determine dT.vi"("error in (no error)"=w361, "Time/Div"=w363, "Program Data"=w362) -> ("error out"=w360:errorcluster, "dT"=w367:dbl, "Program Data Out"=w364:T18)  [unwired: 4 in, 2 out]
            n141 = Bundle By Name(cluster=w364, "Time"=w368, "dT"=w367) -> (w369:T18)
          }
        }
        n142 = call "Load Waveform Parameters.vi"("error in (no error)"=w336, "Program Data"=w344) -> ("error out"=w342:errorcluster, "Program Data Out"=w340:T18)  [unwired: 8 in]
        n143 = call "Idle.vi"("error in (no error)"=w342, "Program Data"=w340) -> ("error out"=w341:errorcluster, "Program Data Out"=w339:T18)  [unwired: 7 in, 1 out]
      }
      frame "Autoscale" {
        w370 = "Volts/Div"
        # "Calculate the best Volts/Div to visualize\nthe signal."
        n144 = call "Autoscale.vi"("error in (no error)"=w380, "Program Data"=w379) -> ("error out"=w374:errorcluster, "CH1 Volts/Div"=w373:T14, "CH0 Volts/Div"=w378:T14, "Program Data Out"=w376:T18)  [unwired: 6 in]
        n145 = property on="Volts/Div" class="Knob (strict)"("Value"=w378) -> ()  [unwired: 2 in, 2 out]
        n146 = property on="Volts/Div" class="Knob (strict)"("Value"=w373) -> ()  [unwired: 2 in, 2 out]
        n147 = call "Channel 0 Selection.vi"("error in (no error)"=w374, "Data"=w370) -> ("error out"=w372:errorcluster)  [unwired: 8 in, 1 out]
        n148 = call "Channel 1 Selection.vi"("error in (no error)"=w372, "Data"=w370) -> ("error out"=w371:errorcluster)  [unwired: 8 in, 1 out]
        n149 = call "Idle.vi"("error in (no error)"=w371, "Program Data"=w376) -> ("error out"=w377:errorcluster, "Program Data Out"=w375:T18)  [unwired: 7 in, 1 out]
      }
      frame "Stop" {
        w381 = T28 {"Acquire?"=FALSE, "Wave Parameters"={"Frequency (Hz)"=0.0, "Phase offset (deg)"=0.0, "Vpeak (V)"=0.0, "Offset (V)"=0.0, "Waveform"=enum."Sine", "Channel"=enum."CH1"}, "Time"={"Time/Div"=9.0}}  # CH1
        # "Tell the myRIO to zero all outputs.\nDisconnect from myRIO.\nEnd program."
        n150 = property on="Time" class="Clust (strict)"() -> ("Value"=w393:T10)  [unwired: 2 in, 2 out]
        n151 = Bundle By Name(cluster=T28 {"Acquire?"=FALSE, "Wave Parameters"={"Frequency (Hz)"=5.0, "Phase offset (deg)"=0.0, "Vpeak (V)"=0.0, "Offset (V)"=0.0, "Waveform"=enum."Sine", "Channel"=enum."CH0"}, "Time"={"Time/Div"=0.0}} ("Params"), "Time"=w393, "Acquire?"=FALSE) -> (w392:T28)
        n152 = Flatten To String(anything=w392, error in (no error)=w391) -> (data string=w389:string, error out=w390:errorcluster)  [unwired: 2 in, 1 out]
        n153 = call "Send Communiation to Target.vi"("error in"=w390, "Data"=w389, "Name"="Params", "Program Data"=w387) -> ("error out"=w382:errorcluster, "Program Data Out"=w383:T18)  [unwired: 6 in]
        n154 = call "Load Waveform Parameters.vi"("error in (no error)"=w382, "Params"=w381, "Program Data"=w383) -> ("error out"=w385:errorcluster, "Program Data Out"=w384:T18)  [unwired: 7 in]
        n155 = call "Disconnect from Target.vi"("error in (no error)"=w385, "Program Data"=w384) -> ("error out"=w388:errorcluster, "Program Data out"=w386:T18)  [unwired: 8 in]
      }
    }
    n156 = Unbundle By Name(w46) -> ("Measurements"=→"Measurements":T6, "FGen.Enable Sweep"=→"Sweep?":bool, "Acquire?"=→"Acquiring?":bool, "FGen.Run"=→"Gen?":bool)
  }
  n157 = while {
    tunnel: w30 -> [w400]
    tunnel: [w399] -> w33
    tunnel: w10 -> [w398]
    stop <- w401 stop-if-true
    # "Event Handler"
    n158 = event shown="[8] \"Time\": Value Change" {
      selector: w398 -> [_ _ _ _ _ _ _ _ _ _]
      dyn-events: _ -> [_ _ _ _ _ _ _ _ _ _]
      timeout: _ -> [_ _ _ _ _ _ _ _ _ _]
      tunnel: [_ w404 TRUE _ _ _ _ _ _ _] -> w401
      tunnel: w400 -> [_ w403 w416 w420 w427 w439 w451 w472 w489 w502]
      tunnel: [_ w402 w415 w419 w425 w438 w450 w471 w490 w501] -> w399
      event Timeout {
        n159 = event-data() -> ()  [unwired: 1 in, 3 out]
      }
      event Menu Selection (User) {
        # "Process Menu Selections"
        n160 = event-data() -> ("ItemTag"=w405:string)  [unwired: 1 in]
        n161 = case shown="\"Exit\"" w405 {
          tunnel: [FALSE TRUE FALSE] -> w404
          tunnel: w403 -> [w406 w409 w413]
          tunnel: [w406 w408 w411] -> w402
          frame "False", Default {
          }
          frame "Exit" {
            n162 = call "Stop.vi"("error in (no error)"=w409) -> ("error out"=w408:errorcluster)  [unwired: 9 in, 1 out]
          }
          frame "Configure" {
            n163 = call "FGen Configuration.vi"("error in (no error)"=w413) -> ("error out"=w412:errorcluster)  [unwired: 10 in]
            n164 = call "Configure FGen.vi"("error in (no error)"=w412) -> ("error out"=w411:errorcluster)  [unwired: 9 in, 1 out]
          }
        }
      }
      event User Event {
        n165 = event-data() -> ()  [unwired: 1 in, 3 out]
        n166 = call "Stop.vi"("error in (no error)"=w416) -> ("error out"=w415:errorcluster)  [unwired: 9 in, 1 out]
      }
      event "Scope Screen": Cursor Move {
        # "Respond to Cursor Move\nUser Event"
        n167 = event-data() -> ("CursRef"=w424:refnum<vi>)  [unwired: 1 in, 2 out]
        n168 = property class="Curs"(reference=w424) -> ("Cursor Name"=w423:string, "Cursor X"=w422:dbl, "Cursor Y"=w421:dbl)  [unwired: 1 in, 2 out]
        n169 = Bundle("Cursor Name"=w423, "Cursor X"=w422, "Cursor Y"=w421) -> (w418:T31)  [unwired: 1 in]
        n170 = call "Update Cursors.vi"("error in (no error)"=w420, "Data"=w418) -> ("error out"=w419:errorcluster)  [unwired: 8 in, 1 out]
      }
      event Value Change {
        # "Process new Options"
        n171 = event-data() -> ("OldVal"=w431:T4, "NewVal"=w430:T4, "CtlRef"=w429:refnum<vi>)  [unwired: 1 in]
        n172 = Not Equal?(x=w431, y=w430) -> (x != y?=w436:T32)
        n173 = property class="Clust (strict)"(reference=w429) -> ("Controls[]"=w428:refnum<vi>[])  [unwired: 1 in, 2 out]
        n174 = Cluster To Array(cluster=w436) -> (array=w435:bool[])
        n175 = Search 1D Array(1D array=w435, element=TRUE) -> (index of element=w433:i32)  [unwired: 1 in]
        n176 = Index Array(array=w428, index=w433) -> (element=w432:refnum<vi>)
        n177 = property class="Ctl"(reference=w432) -> ("Label.Text"=w426:string)  [unwired: 1 in, 2 out]
        n178 = call "Option Selection.vi"("error in (no error)"=w427, "Data"=w426) -> ("error out"=w425:errorcluster)  [unwired: 8 in, 1 out]
      }
      event Value Change {
        # "Process changes to \nChannel 0 Settings"
        n179 = event-data() -> ("OldVal"=w443:T12, "NewVal"=w442:T12, "CtlRef"=w441:refnum<vi>)  [unwired: 1 in]
        n180 = Not Equal?(x=w443, y=w442) -> (x != y?=w448:T33)
        n181 = property class="Clust (strict)"(reference=w441) -> ("Controls[]"=w440:refnum<vi>[])  [unwired: 1 in, 2 out]
        n182 = Cluster To Array(cluster=w448) -> (array=w447:bool[])
        n183 = Search 1D Array(1D array=w447, element=TRUE) -> (index of element=w445:i32)  [unwired: 1 in]
        n184 = Index Array(array=w440, index=w445) -> (element=w444:refnum<vi>)
        n185 = property class="Ctl"(reference=w444) -> ("Label.Text"=w437:string)  [unwired: 1 in, 2 out]
        n186 = call "Channel 0 Selection.vi"("error in (no error)"=w439, "Data"=w437) -> ("error out"=w438:errorcluster)  [unwired: 8 in, 1 out]
      }
      event Value Change {
        # "Process changes to \nChannel 1 Settings"
        n187 = event-data() -> ("OldVal"=w455:T12, "NewVal"=w454:T12, "CtlRef"=w453:refnum<vi>)  [unwired: 1 in]
        n188 = Not Equal?(x=w455, y=w454) -> (x != y?=w460:T33)
        n189 = property class="Clust (strict)"(reference=w453) -> ("Controls[]"=w452:refnum<vi>[])  [unwired: 1 in, 2 out]
        n190 = Cluster To Array(cluster=w460) -> (array=w459:bool[])
        n191 = Search 1D Array(1D array=w459, element=TRUE) -> (index of element=w457:i32)  [unwired: 1 in]
        n192 = Index Array(array=w452, index=w457) -> (element=w456:refnum<vi>)
        n193 = property class="Ctl"(reference=w456) -> ("Label.Text"=w449:string)  [unwired: 1 in, 2 out]
        n194 = call "Channel 1 Selection.vi"("error in (no error)"=w451, "Data"=w449) -> ("error out"=w450:errorcluster)  [unwired: 8 in, 1 out]
      }
      event Value Change {
        # "Determine which Acuisition option\nwas selected and process."
        n195 = event-data() -> ("OldVal"=w469:T8, "NewVal"=w468:T8, "CtlRef"=w470:refnum<vi>)  [unwired: 1 in]
        n196 = Not Equal?(x=w469, y=w468) -> (x != y?=w467:T34)
        n197 = property class="Clust"(reference=w470) -> ("Controls[]"=w464:refnum<vi>[])  [unwired: 1 in, 2 out]
        n198 = Cluster To Array(cluster=w467) -> (array=w466:bool[])
        n199 = Search 1D Array(1D array=w466, element=TRUE) -> (index of element=w463:i32)  [unwired: 1 in]
        n200 = Index Array(array=w464, index=w463) -> (element=w462:refnum<vi>)
        n201 = property class="Ctl"(reference=w462) -> ("Label.Text"=w461:string)  [unwired: 1 in, 2 out]
        n202 = case shown="\"Acquire\"" w461 {
          tunnel: w472 -> [w473 w479 w485 w487]
          tunnel: [w473 w476 w484 w486] -> w471
          frame "False", Default {
          }
          frame "Acquire" {
            n203 = property on="Acquisition Mode" class="Enum (strict)"(error in=w479) -> (error out=w478:errorcluster, "Value"=w477:T9)  [unwired: 1 in, 1 out]
            n204 = case shown="\"Run Once\"" w477 {
              tunnel: w478 -> [w481 w483]
              tunnel: [w481 w483] -> w475
              tunnel: [TRUE FALSE] -> w474
              frame "Run Continuously", Default {
              }
              frame "Run Once" {
              }
            }
            n205 = call "Start Scope Acquire.vi"("error in (no error)"=w475, "Continuous?"=w474) -> ("error out"=w476:errorcluster)  [unwired: 8 in, 1 out]
          }
          frame "Stop" {
            n206 = call "Stop Scope Acquire.vi"("error in (no error)"=w485) -> ("error out"=w484:errorcluster)  [unwired: 9 in, 1 out]
          }
          frame "Autoscale" {
            n207 = call "Auto Scale.vi"("error in (no error)"=w487) -> ("error out"=w486:errorcluster)  [unwired: 9 in, 1 out]
          }
        }
      }
      event Value Change {
        # "Notify Processing to \nuse new Time settings."
        n208 = event-data() -> ()  [unwired: 1 in, 1 out]
        n209 = call "Time Div.vi"("error in (no error)"=w489, "Data"="Time") -> ("error out"=w490:errorcluster)  [unwired: 8 in, 1 out]
      }
      event Value Change {
        # "Notify Processing to act on button press."
        n210 = event-data() -> ("OldVal"=w499:T1, "NewVal"=w498:T1, "CtlRef"=w500:refnum<vi>)  [unwired: 1 in]
        n211 = Not Equal?(x=w499, y=w498) -> (x != y?=w497:T35)
        n212 = property class="Clust"(reference=w500) -> ("Controls[]"=w494:refnum<vi>[])  [unwired: 1 in, 2 out]
        n213 = Cluster To Array(cluster=w497) -> (array=w496:bool[])
        n214 = Search 1D Array(1D array=w496, element=TRUE) -> (index of element=w493:i32)  [unwired: 1 in]
        n215 = Index Array(array=w494, index=w493) -> (element=w492:refnum<vi>)
        n216 = property class="Ctl"(reference=w492) -> ("Label.Text"=w491:string)  [unwired: 1 in, 2 out]
        n217 = case shown="\"Stop\"" w491 {
          tunnel: w502 -> [w503 w505 w506]
          tunnel: [w503 w504 w507] -> w501
          frame "False", Default {
          }
          frame "Generate" {
            n218 = call "Start FGen.vi"("error in (no error)"=w505) -> ("error out"=w504:errorcluster)  [unwired: 9 in, 1 out]
          }
          frame "Stop" {
            n219 = call "Stop FGen.vi"("error in (no error)"=w506) -> ("error out"=w507:errorcluster)  [unwired: 9 in, 1 out]
          }
        }
      }
    }
  }
  n220 = Merge Errors(w33, w32) -> (w8:errorcluster)
  n221 = call "User Event FGV.vi"("Action"=User_Event_Action_Enum."Destroy", "error in (no error)"=w8) -> ("error out"=w9:errorcluster)  [unwired: 8 in, 1 out]
  n222 = call "Release Desktop Queue.vi"("error in (no error)"=w9) -> ("error out"=→"error out":errorcluster)  [unwired: 10 in]
